vi "RM.setDeviceReservationDB.vi"(8 "error in":errorcluster, 9 "reservation DB in":variant, 10 "device name":string="deviceName", 11 "Item Ref in":T1 format="%.0x") -> (0 "error out":errorcluster, 1 "replaced":bool, 3 "Item Ref out":T1 format="%.0x")   [LabVIEW 2016, in "FPGA Addon Shared.lvlib"]
uses:
  FPGA Addon Shared.lvlib
  <vilib>/NI Veristand/Custom Device API/Custom Device Item Ref.ctl
  <vilib>/NI Veristand/Custom Device API/Get Item Property (Variant).vi
  <vilib>/NI Veristand/Custom Device API/Set Item Property (Variant).vi
  <vilib>/NI VeriStand/Custom Device Tools/Custom Device Utility Library/Custom Device Utility Library.lvlib
  <vilib>/NI VeriStand/Custom Device API/Custom Device API.lvlib
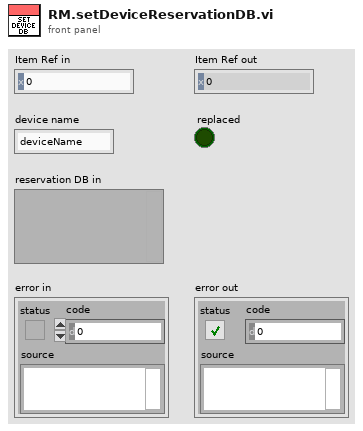
[diagram p1: front panel]
types:
  T1 = typedef "Custom Device API.lvlib/Custom Device Item Ref.ctl" = u64
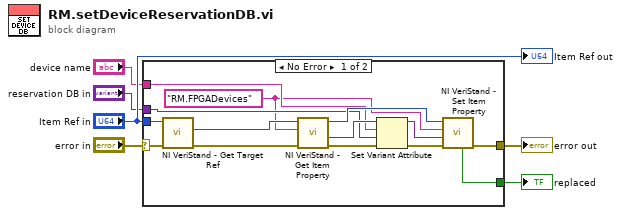
[diagram p0: block diagram]
diagram:
  n1 = case shown="No Error" "error in" {
    selector: "error in" -> [w19 w21]
    tunnel: "Item Ref in" -> [w20 _]
    tunnel: [w17 _] -> w6
    tunnel: [w18 w21] -> w4
    tunnel: "device name" -> [w12 _]
    tunnel: "reservation DB in" -> [w13 _]
    frame No Error {
      w7 = "RM.FPGADevices" ("Property Name")
      n2 = call <vilib>:"NI VeriStand - Get Target Ref.vi"("error in"=w19, "Item Ref in"=w20) -> ("error out"=w10:errorcluster, "Target Ref"=w16:T1)  [unwired: 6 in, 2 out]
      n3 = call-poly <vilib>:"NI VeriStand - Get Item Property.vi"("error in (no error)"=w10, "Property Name"=w7, "Item Ref in"=w16) -> ("error out"=w9:errorcluster, "Value"=w14:variant, "Item Ref out"=w15:T1)  [unwired: 5 in, 1 out]
      n4 = Set Variant Attribute(Variant=w14, name=w12, value=w13, error in=w9) -> (Variant out=w11:variant, error out=w8:errorcluster)  [unwired: 1 out]
      n5 = call-poly <vilib>:"NI VeriStand - Set Item Property.vi"("error in (no error)"=w8, "Value"=w11, "Property Name"=w7, "Item Ref in"=w15) -> ("error out"=w18:errorcluster, "Replaced"=w17:bool)  [unwired: 5 in, 1 out]
    }
    frame Error {
    }
  }
  "replaced" <- w6
  "error out" <- w4
  "Item Ref out" <- "Item Ref in"
